vi "Configure Sparse Marker [SM] Core.vi"(5 "Destination Terminal (None)":string(combo) caption="destination terminal (None)", 6 "Indexes Array":i64[](array[numeric]) caption="indexes array", 7 "Number Indexes":i64 caption="number indexes" format="%.0g", 8 "error in (no error)":errorcluster, 9 "Waveform Handle":i32 caption="waveform handle" format="%.0g", 10 "Marker Name (\"\")":string caption="marker name (\"\")", 11 "CS++Fgen in":refnum<class "CS++Fgen.lvclass">) -> (0 "error out":errorcluster, 3 "CS++Fgen out":refnum<class "CS++Fgen.lvclass">)   [LabVIEW 2013, in "CS++Fgen.lvlib" / "CS++Fgen.lvclass"]
doc: "This VI configures the common sparse marker properties. These properties are the sparse marker waveform handle and destination.\n \nThis VI also configures which waveform and sample number the output is associated with.\n\nNote:\n\n(1) This VI is part of the IviFgenSparseMarker [SM] extension group."
uses:
  CS++Fgen.lvclass
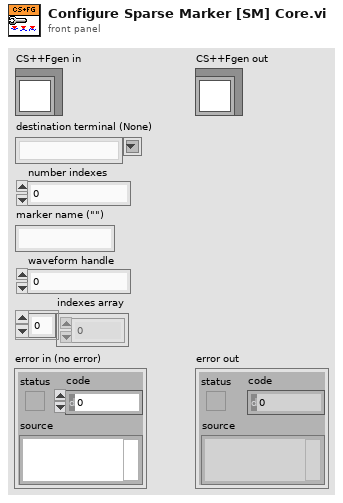
[diagram p1: front panel]
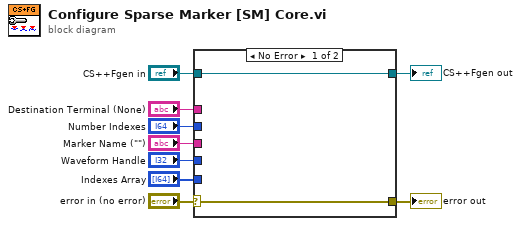
[diagram p0: block diagram]
diagram:
  n1 = case shown="No Error" "error in (no error)" {
    selector: "error in (no error)" -> [w10 w13]
    tunnel: [w10 w13] -> w8
    tunnel: [w11 w12] -> w6
    tunnel: "CS++Fgen in" -> [w11 w12]
    tunnel: "Marker Name (\"\")" -> [_ _]
    tunnel: "Destination Terminal (None)" -> [_ _]
    tunnel: "Number Indexes" -> [_ _]
    tunnel: "Waveform Handle" -> [_ _]
    tunnel: "Indexes Array" -> [_ _]
    frame No Error {
    }
    frame Error {
    }
  }
  "error out" <- w8
  "CS++Fgen out" <- w6
